vi "Write Value.vi"(8 "error in (no error)":errorcluster, 10 "Data":string, 11 "String in":refnum<class "Const_Str.lvclass">) -> (0 "error out":errorcluster, 3 "String out":refnum<class "Const_Str.lvclass">)   [LabVIEW 2021, in "Const_Str.lvclass"]
uses:
  Const_Str.lvclass
  Const_Str.lvclass/Const_Str.ctl
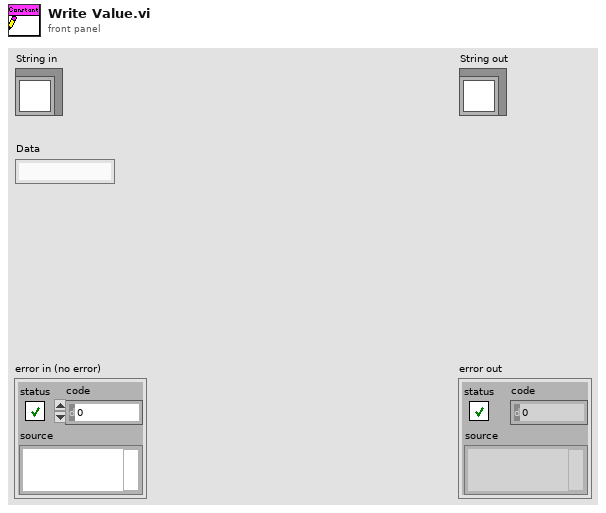
[diagram p1: front panel]
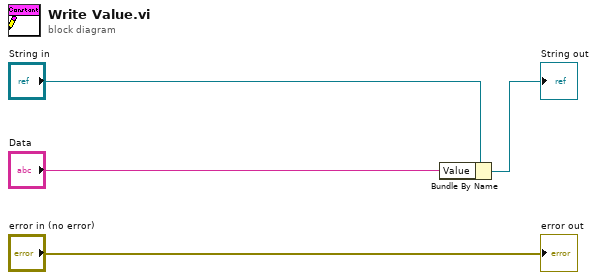
[diagram p0: block diagram]
diagram:
  n1 = Bundle By Name(cluster="String in", "Value"="Data") -> (→"String out":refnum<class "Const_Str.lvclass">)
  "error out" <- "error in (no error)"
